vi "Set Number of Test Methods.vi"(8 "error in (no error)":errorcluster, 10 "Method Count":u32, 11 "Result Table.lvclass":refnum<class "Result Table V2.lvclass">) -> (0 "error out":errorcluster, 3 "Result Table":refnum<class "Result Table V2.lvclass">)   [LabVIEW 2020, in "Result Table V2.lvclass"]
uses:
  Result Table V2.lvclass
  Result Table V2.lvclass/Result Table V2.ctl
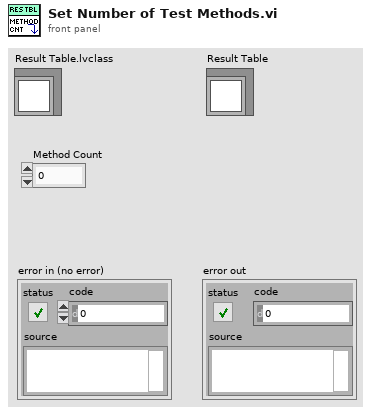
[diagram p1: front panel]
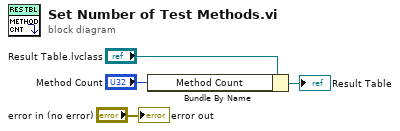
[diagram p0: block diagram]
diagram:
  n1 = Bundle By Name(cluster="Result Table.lvclass", "Method Count"="Method Count") -> (→"Result Table":refnum<class "Result Table V2.lvclass">)
  "error out" <- "error in (no error)"
